vi "IntakeDefaultForward.vi"   [LabVIEW 2014, in "IntakeLib.lvlib"]
uses:
  IntakeLib.lvlib
  <vilib>/Rock Robotics/WPI/Solenoid/WPI_SolenoidValue.ctl
types:
  T1 = typedef "WPI_SolenoidValue.ctl" = enum16{"Off", "On", "Forward", "Reverse"}
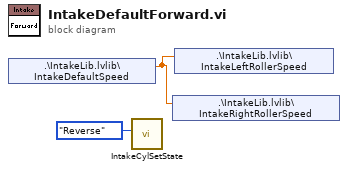
[diagram p0: block diagram]
diagram:
  n1 = shared-variable ".\\IntakeLib.lvlib\\IntakeDefaultSpeed"() -> (w1:dbl)  [unwired: 1 in, 1 out]
  n2 = call "IntakeCylSetState.vi"("IntakeCylState"=WPI_SolenoidValue."Reverse") -> ()  [unwired: 11 in]
  n3 = shared-variable ".\\IntakeLib.lvlib\\IntakeRightRollerSpeed"(w1) -> ()  [unwired: 1 in, 1 out]
  n4 = shared-variable ".\\IntakeLib.lvlib\\IntakeLeftRollerSpeed"(w1) -> ()  [unwired: 1 in, 1 out]
